vi "Control.vi"() -> ()   [LabVIEW 2018]
uses:
  <vilib>/Utility/file.llb/Read Delimited Spreadsheet (string).vi
panel:
  in  "Array":string[](array[string])
  out "Projects":string[](array[string])
  in  "File Information":T1={"Ring"=0, "SubFolder"="Temp Dependence", "Filename (Meas. Description)"="200C", "Measurement number"=2} {"Ring" items=["H2DT", "VaporTubes", "MaterialsTesting", "ThermalCond", "SeedFeeder", "Rando"]}
  in  "Path":path=path "C:/Users/bowenm/Documents/ProjectIndex.csv"
  in  "?":bool
  in  "File Close Action":enum16{"Prompt", "Keep", "Archive", "Trash"}(ring)
  in  "Wait time (ms)":i32=250
  in  "Vi Selection":bool[](array[boolean])=[TRUE, TRUE, TRUE, TRUE, FALSE]
  in  "Measuring":bool=TRUE
  # "Spectrometer"
  # "Sensors"
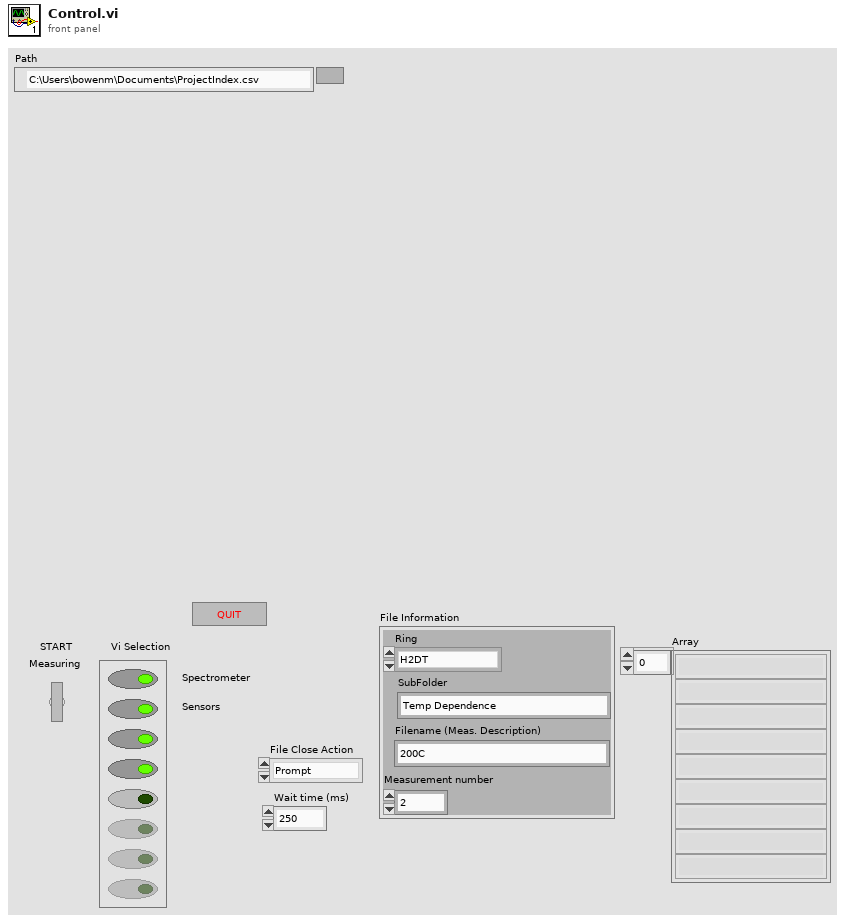
[diagram p1: front panel]
types:
  T1 = cluster{"Ring":u16, "SubFolder":string, "Filename (Meas. Description)":string, "Measurement number":i32}
  T2 = enum32{"Invalid", "Standard", "Closed", "Hidden", "Minimized", "Maximized"}
  T3 = enum32{"Bad", "Idle", "Run top level", "Running"}
  T4 = cluster{"Project":u16, "SubFolder":string, "Filename (Meas. Description)":string, "Measurement number":i32}
  T5 = cluster{"VI out":refnum<vi>, "error out":errorcluster, "Output cluster refnum":refnum<vi>, enum16{"TestVi", "TestVi_2", "TestVi_3"}}
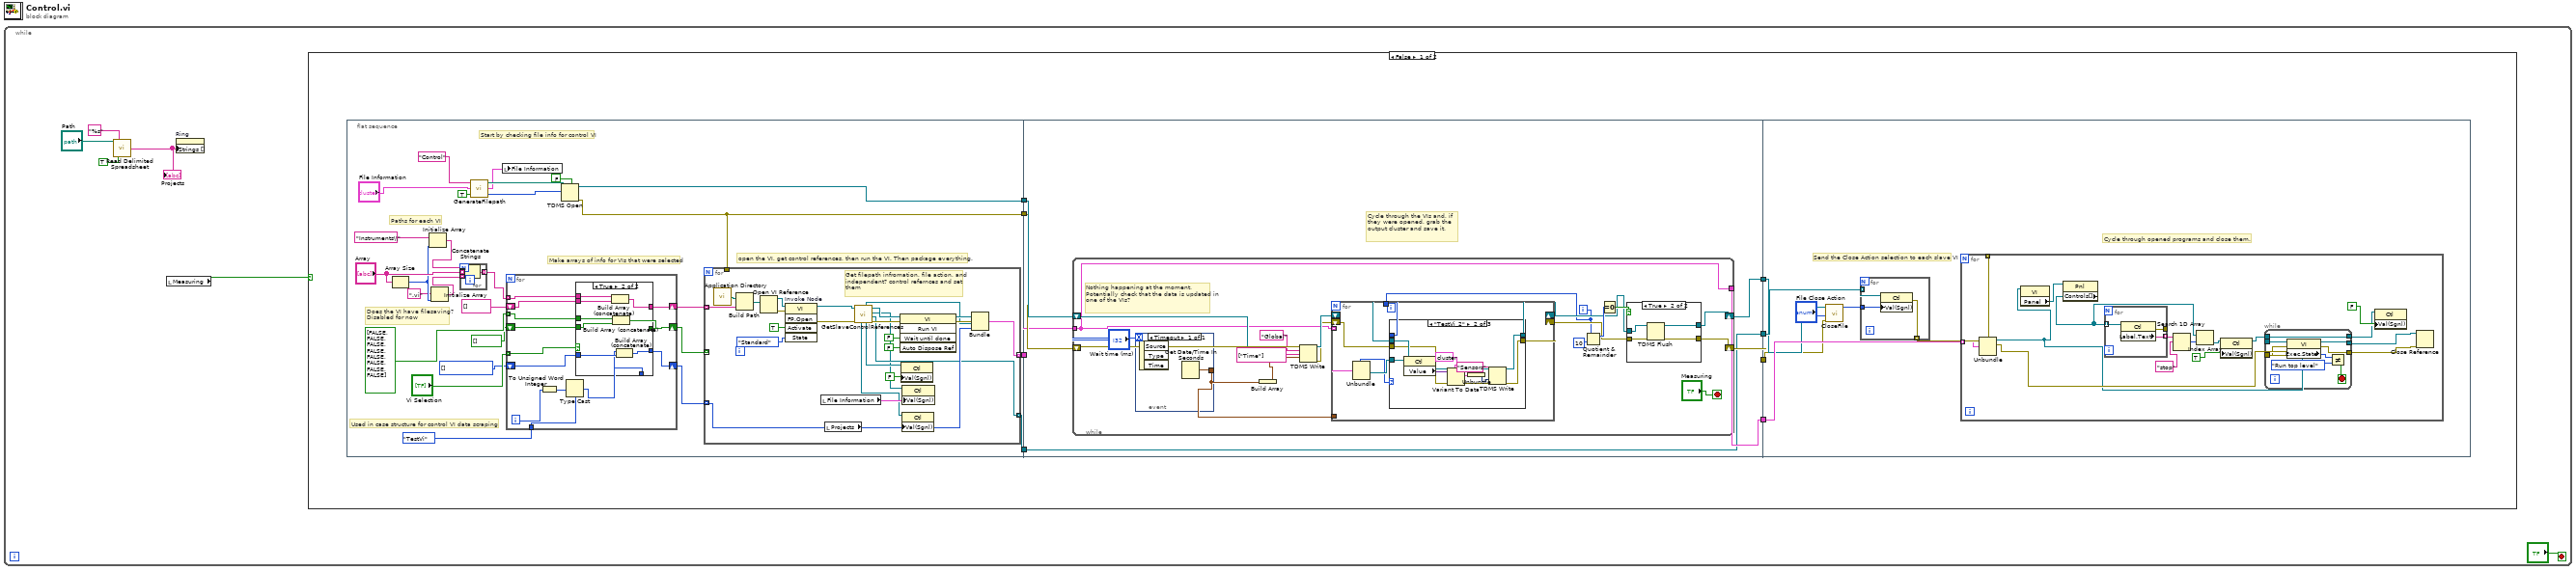
[diagram p0: block diagram]
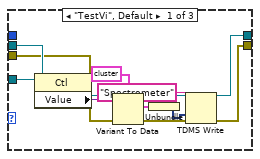
[diagram p3: hidden frame]
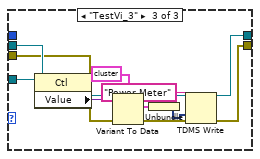
[diagram p4: hidden frame]
diagram:
  n1 = while {
    stop <- "?" stop-if-true
    n2 = call-poly <vilib>:"Read Delimited Spreadsheet.vi"("file path (dialog if empty)"="Path", "format (%s)"="%s", "transpose? (F)"=TRUE) -> ("first row"=w4:string[])  [unwired: 7 in, 5 out]
    "Projects" <- w4
    n3 = local read "Measuring"() -> (w6:bool)
    n4 = property on="Ring" class="Ring (strict)"("Strings []"=w4) -> ()  [unwired: 2 in, 2 out]
    n5 = case shown="False" w6 {
      frame False {
        n6 = flat-sequence {
          tunnel: [w26] -> w14
          tunnel: [w23] -> w13
          tunnel: [w32] -> w12
          tunnel: [w25] -> w11
          tunnel: [w101] -> w10
          tunnel: [w102] -> w9
          tunnel: [w97] -> w8
          tunnel: w14 -> [w100]
          tunnel: w13 -> [w99]
          tunnel: w12 -> [w98]
          tunnel: [w96] -> w7
          tunnel: w11 -> [w96]
          tunnel: w10 -> [w168]
          tunnel: w9 -> [w169]
          tunnel: w8 -> [w173]
          tunnel: w7 -> [w171]
          frame #0 {
            w33 = enum16{"TestVi", "TestVi_2", "TestVi_3"}[] [] items=["TestVi", "TestVi_2", "TestVi_3"]
            # "Start by checking file info for control VI"
            # "open the VI, get control references, then run the VI. Then package everything."
            # "Make arrays of info for VIs that were selected"
            # "Paths for each VI"
            # "Does the VI have filesaving?\nDisabled for now"
            # "Used in case structure for control VI data scraping"
            n7 = Array Size(array="Array") -> (size(s)=w20:i32)
            n8 = Initialize Array("Instruments\\" ("string"), w20) -> (w18:string[])
            n9 = Initialize Array(".vi" ("string"), w20) -> (w19:string[])
            n10 = for {
              tunnel: w18 -> [w45] mode=indexing
              tunnel: w19 -> [w44] mode=indexing
              tunnel: "Array" -> [w43] mode=indexing
              tunnel: [w42] -> w15 mode=indexing
              n11 = Concatenate Strings(w45, w43, w44) -> (w42:string)
            }
            n12 = call "GenerateFilepath.vi"("Check for file?"=TRUE, "File Information"="File Information", "Instrument"="Control") -> ("File Action"=w30:i32, "File Information Out"=w29:T4, "File Path Out"=w31:path)
            n13 = local write "File Information"(w29) -> ()
            n14 = for {
              tunnel: bool[] [FALSE, FALSE, FALSE, FALSE, FALSE, FALSE, FALSE, FALSE] ("Vi Selection 2") -> [w54] mode=indexing
              tunnel: "Vi Selection" -> [w55] mode=indexing
              tunnel: w15 -> [w51] mode=indexing
              tunnel: enum16{"TestVi", "TestVi_2", "TestVi_3"}."TestVi" -> [w57]
              shift-right: [w53] -> w40
              shift-left: bool[] [] -> [w52]
              shift-right: [w50] -> w39
              shift-left: string[] [] -> [w49]
              shift-right: [w47] -> w41
              shift-left: w33 -> [w46]
              i -> [w56]
              n15 = To Unsigned Word Integer(number=w56) -> (unsigned 16bit integer=w58:u16)
              n16 = Type Cast(type=w57, x=w58) -> (*(type *) &x=w48:enum16{"TestVi", "TestVi_2", "TestVi_3"})
              n17 = case shown="True" w55 {
                tunnel: w54 -> [_ w70]
                tunnel: [w61 w69] -> w53
                tunnel: w52 -> [w61 w68]
                tunnel: w51 -> [_ w67]
                tunnel: [w60 w66] -> w50
                tunnel: w49 -> [w60 w65]
                tunnel: w48 -> [_ w63]
                tunnel: [w59 w62] -> w47
                tunnel: w46 -> [w59 w64]
                frame False {
                }
                frame True {
                  n18 = Build Array (concatenate)(w67, w65) -> (w66:string[])
                  n19 = Build Array (concatenate)(w70, w68) -> (w69:bool[])
                  n20 = Build Array (concatenate)(w63, w64) -> (w62:enum16{"TestVi", "TestVi_2", "TestVi_3"}[])
                }
              }
            }
            n21 = TDMS Open(5:FALSE ("create index file? (T)"), 10:w30, 11:w31) -> (0:w23:errorcluster, 3:w26:refnum<k34>)  [unwired: 4 in]
            n22 = for {
              tunnel: w39 -> [w95] mode=indexing
              tunnel: w40 -> [_] mode=indexing
              tunnel: [w88] -> w32 mode=indexing
              tunnel: w41 -> [w81] mode=indexing
              tunnel: [w80] -> w25 mode=indexing
              tunnel: w23 -> [_]
              # "Get filepath infromation, file action, and independent? control refernces and set them"
              n23 = call <vilib>:"Application Directory.vi"() -> ("Application Directory"=w93:path)
              n24 = Build Path(base path=w93, name or relative path=w95) -> (appended path=w91:path)
              n25 = Open VI Reference(vi path=w91) -> (vi reference=w94:refnum<vi>, error out=w92:errorcluster)  [unwired: 5 in]
              n26 = invoke on="Invoke Node" class="VI" method="FP.Open"(reference=w94, error in=w92, "Activate"=TRUE ("Activate?"), "State"=T2."Standard") -> (reference out=w83:refnum<vi>, error out=w82:errorcluster)  [unwired: 1 in, 3 out]
              n27 = local read "File Information"() -> (w78:T1)
              n28 = local read "Projects"() -> (w72:string[])
              n29 = call "GetSlaveControlReferences.vi"("error in (no error)"=w82, "VI in"=w83) -> ("error out"=w86:errorcluster, "File Close Action Refnum"=w80:refnum<vi>, "File info Refnum"=w73:refnum<vi>, "VI out"=w87:refnum<vi>, "Indepedent? Control"=w77:refnum<vi>, "Output cluster refnum"=w79:refnum<vi>, "Project Refnum"=w71:refnum<vi>)  [unwired: 3 in]
              n30 = invoke class="VI" method="Run VI"(reference=w87, error in=w86, "Wait until done"=FALSE ("Wait Until Done"), "Auto Dispose Ref"=FALSE ("Auto Dispose Reference")) -> (reference out=w90:refnum<vi>, error out=w89:errorcluster)  [unwired: 1 in, 3 out]
              n31 = property class="Ctl"(reference=w77, "Val(Sgnl)"=FALSE) -> ()  [unwired: 1 in, 2 out]
              n32 = property class="Ctl"(reference=w71, "Val(Sgnl)"=w72) -> ()  [unwired: 1 in, 2 out]
              n33 = property class="Ctl"(reference=w73, "Val(Sgnl)"=w78) -> ()  [unwired: 1 in, 2 out]
              n34 = Bundle("VI out"=w90, "error out"=w89, "Output cluster refnum"=w79, w81) -> (w88:T5)  [unwired: 1 in]
            }
          }
          frame #1 {
            # "Cycle through the VIs and, if they were opened, grab the output cluster and save it."
            n35 = while {
              shift-right: [w103] -> w102
              shift-left: w100 -> [w115]
              shift-right: [w109] -> w101
              shift-left: w99 -> [w116]
              tunnel: w98 -> [w104]
              tunnel: [w104] -> w97
              i -> [w105]
              stop <- "Measuring" stop-if-true
              # "Nothing happening at the moment. Potentially check that the data is updated in one of the VIs?"
              n36 = event shown="[0] Timeout" {
                selector: _ -> [_]
                dyn-events: _ -> [_]
                timeout: "Wait time (ms)" -> [_]
                tunnel: [w122] -> w107
                event Timeout {
                  n37 = event-data() -> ()  [unwired: 1 in, 3 out]
                  n38 = Get Date/Time In Seconds() -> (seconds since 1Jan1904=w122:timestamp)
                }
              }
              n39 = Build Array(w107) -> (w114:timestamp[])
              n40 = TDMS Write(0:w115, 5:"Global" ("group name in (Untitled)"), 7:string[] ["Time"] ("channel name(s) in (Untitled)"), 9:w114, 11:w116) -> (4:w111:refnum<k34>, 15:w110:errorcluster)  [unwired: 1 in, 2 out]
              n41 = for {
                tunnel: w104 -> [w130] mode=indexing
                shift-right: [w127] -> w118
                shift-left: w111 -> [w129]
                shift-right: [w126] -> w108
                shift-left: w110 -> [w128]
                tunnel: w107 -> [_]
                tunnel: w105 -> [w123]
                n42 = Unbundle(w130) -> ("Output cluster refnum"=w125:refnum<vi>, w124:enum16{"TestVi", "TestVi_2", "TestVi_3"})  [unwired: 2 out]
                n43 = case shown="\"TestVi_2\"" w124 {
                  tunnel: w125 -> [w139 w149 w159]
                  tunnel: w129 -> [w138 w148 w158]
                  tunnel: w128 -> [w135 w145 w155]
                  tunnel: [w136 w146 w156] -> w127
                  tunnel: [w134 w144 w154] -> w126
                  tunnel: w123 -> [_ _ _]
                  frame "TestVi", Default {
                    n44 = property class="Ctl"(reference=w139) -> ("Value"=w140:variant)  [unwired: 1 in, 2 out]
                    n45 = Variant To Data(type=cluster{"Sine with Uniform Noise":dynamicdata} {"Sine with Uniform Noise"=[{"t0"=timestamp(3610577859.0026608 s since 1904-01-01), "dt"=0.001, "Y"=[-0.16133839886461693], "attributes"=variant("NI_ChannelName"=variant(string "Sine with Uniform Noise"), "NI_ExpIsRelativeTime"=variant(bool FALSE), "NI_ExpStartTimeStamp"=variant(timestamp timestamp(3610577841.968661 s since 1904-01-01)), "NI_ExpTimeStamp"=variant(timestamp timestamp(3610577859.0026608 s since 1904-01-01)), "NI_ExpXDimension"=variant(string "t"))}]} ("output cluster"), Variant=w140) -> (data=w133:cluster{"Sine with Uniform Noise":dynamicdata})  [unwired: 1 in, 1 out]
                    n46 = Unbundle(w133) -> ("Sine with Uniform Noise"=w132:dynamicdata)
                    n47 = TDMS Write(0:w138, 5:"Spectrometer" ("group name in (Untitled)"), 9:w132, 11:w135) -> (4:w136:refnum<k34>, 15:w134:errorcluster)  [unwired: 2 in, 2 out]
                  }
                  frame "TestVi_2" {
                    n48 = property class="Ctl"(reference=w149) -> ("Value"=w150:variant)  [unwired: 1 in, 2 out]
                    n49 = Variant To Data(type=cluster{"Sine with Uniform Noise":dynamicdata} {"Sine with Uniform Noise"=[{"t0"=timestamp(3610577859.0026608 s since 1904-01-01), "dt"=0.001, "Y"=[-0.16133839886461693], "attributes"=variant("NI_ChannelName"=variant(string "Sine with Uniform Noise"), "NI_ExpIsRelativeTime"=variant(bool FALSE), "NI_ExpStartTimeStamp"=variant(timestamp timestamp(3610577841.968661 s since 1904-01-01)), "NI_ExpTimeStamp"=variant(timestamp timestamp(3610577859.0026608 s since 1904-01-01)), "NI_ExpXDimension"=variant(string "t"))}]} ("output cluster"), Variant=w150) -> (data=w143:cluster{"Sine with Uniform Noise":dynamicdata})  [unwired: 1 in, 1 out]
                    n50 = Unbundle(w143) -> ("Sine with Uniform Noise"=w142:dynamicdata)
                    n51 = TDMS Write(0:w148, 5:"Sensors" ("group name in (Untitled)"), 9:w142, 11:w145) -> (4:w146:refnum<k34>, 15:w144:errorcluster)  [unwired: 2 in, 2 out]
                  }
                  frame "TestVi_3" {
                    n52 = property class="Ctl"(reference=w159) -> ("Value"=w160:variant)  [unwired: 1 in, 2 out]
                    n53 = Variant To Data(type=cluster{"Sine with Uniform Noise":dynamicdata} {"Sine with Uniform Noise"=[{"t0"=timestamp(3610577859.0026608 s since 1904-01-01), "dt"=0.001, "Y"=[-0.16133839886461693], "attributes"=variant("NI_ChannelName"=variant(string "Sine with Uniform Noise"), "NI_ExpIsRelativeTime"=variant(bool FALSE), "NI_ExpStartTimeStamp"=variant(timestamp timestamp(3610577841.968661 s since 1904-01-01)), "NI_ExpTimeStamp"=variant(timestamp timestamp(3610577859.0026608 s since 1904-01-01)), "NI_ExpXDimension"=variant(string "t"))}]} ("output cluster"), Variant=w160) -> (data=w153:cluster{"Sine with Uniform Noise":dynamicdata})  [unwired: 1 in, 1 out]
                    n54 = Unbundle(w153) -> ("Sine with Uniform Noise"=w152:dynamicdata)
                    n55 = TDMS Write(0:w158, 5:"Power Meter" ("group name in (Untitled)"), 9:w152, 11:w155) -> (4:w156:refnum<k34>, 15:w154:errorcluster)  [unwired: 2 in, 2 out]
                  }
                }
              }
              n56 = Quotient & Remainder(x=w105, y=10) -> (x-y*floor(x/y)=w119:i32)  [unwired: 1 out]
              n57 = Equal To 0?(x=w119) -> (x = 0?=w120:bool)
              n58 = case shown="True" w120 {
                tunnel: [w161 w166] -> w103
                tunnel: [w162 w165] -> w109
                tunnel: w108 -> [w162 w164]
                tunnel: w118 -> [w161 w163]
                frame False {
                }
                frame True {
                  n59 = TDMS Flush(4:w164, 7:w163) -> (0:w165:errorcluster, 3:w166:refnum<k34>)
                }
              }
            }
          }
          frame #2 {
            # "Send the Close Action selection to each slave VI"
            # "Cycle through opened programs and close them."
            n60 = call "CloseFile.vi"("error in (no error)"=w168, "Action"="File Close Action", "Refnum in"=w169) -> ("File Close action out"=w167:enum16{"Prompt", "Keep", "Archive", "Trash"})  [unwired: 8 in]
            n61 = for {
              tunnel: w171 -> [w176] mode=indexing
              tunnel: [w175] -> w170 mode=indexing
              tunnel: w167 -> [w174]
              n62 = property class="Ctl"(reference=w176, "Val(Sgnl)"=w174) -> (error out=w175:errorcluster)  [unwired: 1 in, 1 out]
            }
            n63 = for {
              tunnel: w173 -> [w190] mode=indexing
              tunnel: w170 -> [_] mode=indexing
              n64 = Unbundle(w190) -> ("VI out"=w178:refnum<vi>, "error out"=w189:errorcluster)  [unwired: 2 out]
              n65 = property class="VI"(reference=w178) -> ("Panel"=w179:refnum<vi>)  [unwired: 1 in, 2 out]
              n66 = property class="Pnl"(reference=w179) -> ("Controls[]"=w177:refnum<vi>[])  [unwired: 1 in, 2 out]
              n67 = for {
                tunnel: w177 -> [w194] mode=indexing
                tunnel: [w193] -> w186 mode=indexing
                tunnel: [w192] -> _
                n68 = property class="Ctl"(reference=w194) -> (error out=w192:errorcluster, "Label.Text"=w193:string)  [unwired: 1 in, 1 out]
              }
              n69 = Search 1D Array(1D array=w186, element="stop") -> (index of element=w185:i32)  [unwired: 1 in]
              n70 = Index Array(array=w177, index=w185) -> (element=w187:refnum<vi>)
              n71 = property class="Ctl"(reference=w187, "Val(Sgnl)"=TRUE) -> (reference out=w182:refnum<vi>)  [unwired: 1 in, 1 out]
              n72 = while {
                tunnel: w178 -> [w202]
                tunnel: [w201] -> w191
                tunnel: w189 -> [w197]
                tunnel: [w196] -> w188
                tunnel: [w195] -> _
                tunnel: w182 -> [w195]
                tunnel: [w195] -> w180
                stop <- w200 stop-if-true
                n73 = property class="VI"(reference=w202, error in=w197) -> (reference out=w201:refnum<vi>, error out=w196:errorcluster, "Exec.State"=w199:T3)
                n74 = Not Equal?(x=w199, y=T3."Run top level" ("Execution:State 2")) -> (x != y?=w200:bool)
              }
              n75 = property class="Ctl"(reference=w180, "Val(Sgnl)"=FALSE) -> ()  [unwired: 1 in, 2 out]
              n76 = Close Reference(reference=w191, error in (no error)=w188) -> ()  [unwired: 1 out]
            }
          }
        }
      }
      frame True {
      }
    }
  }
